vi "2DGaussianRotationModel.vi"(3 "output control":T1, 4 "data":T2, 5 "X":dbl[](array[numeric]), 6 "a":dbl[](array[numeric])) -> (0 "error out":errorcluster, 1 "f'(X,a)":dbl[][](array[numeric]), 2 "f(X,a)":dbl[](array[numeric]))   [LabVIEW 2015]
doc: "This template is the starting point for creating a model function to be passed to the Nonlinear Curve Fit.vi."
uses:
  <vilib>/gmath/NumericalOptimization/objective function data.ctl
  <vilib>/gmath/NumericalOptimization/LM_output select.ctl
  <vilib>/Analysis/baseanly.llb/A x Vector.vi
  <vilib>/Analysis/Matrix/Numeric/Conversions/Array To Matrix - RA2.vi
  <vilib>/Analysis/NI_AALBase.lvlib
  <vilib>/Analysis/Matrix/NI_Matrix.lvlib
  <vilib>/gmath/NI_Gmath.lvlib
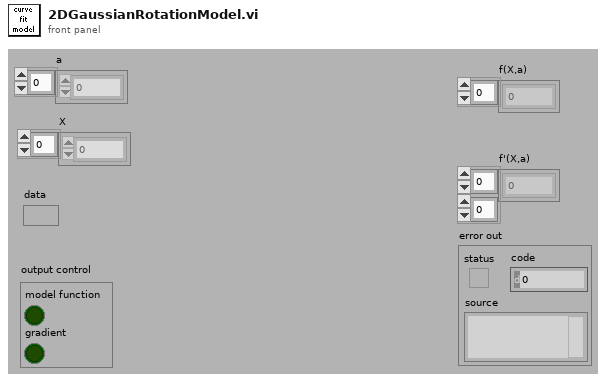
[diagram p1: front panel]
types:
  T1 = typedef "NI_Gmath.lvlib/LM_output select.ctl" = cluster{"model function":bool, "gradient":bool}
  T2 = typedef "NI_Gmath.lvlib/objective function data.ctl" = variant
  T3 = typedef "NI_Matrix.lvlib/RealMatrix.ctl" = dbl[][]
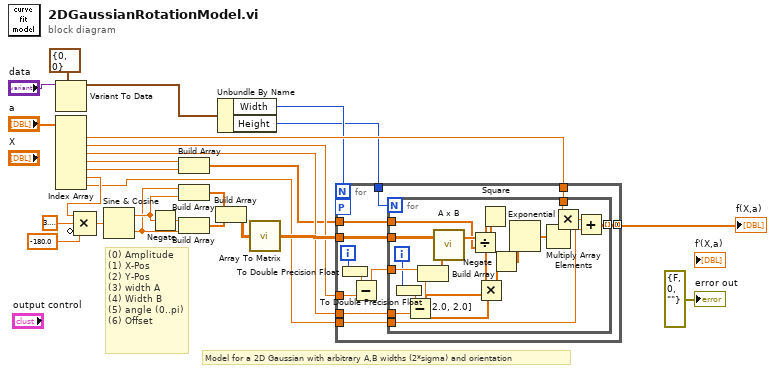
[diagram p0: block diagram]
diagram:
  # "Model for a 2D Gaussian with arbitrary A,B widths (2*sigma) and orientation"
  # "(0) Amplitude\n(1) X-Pos\n(2) Y-Pos\n(3) width A\n(4) Width B\n(5) angle (0..pi)\n(6) Offset"
  n1 = Variant To Data(type=cluster{"Width":i32, "Height":i32} {"Width"=0, "Height"=0} ("Plot Area:Size"), Variant="data") -> (data=w15:cluster{"Width":i32, "Height":i32})  [unwired: 1 in, 1 out]
  n2 = Index Array(array="a") -> (element #1=w19:dbl, element #2=w10:dbl, element #3=w9:dbl, element #4=w18:dbl, element #5=w17:dbl, element #6=w5:dbl, element #7=w4:dbl)  [unwired: 7 in]
  n3 = Compound Arithmetic op=MULTIPLY(w5, 3.141592653589793, invert -180.0 ("value")) -> (w8:dbl)
  n4 = Sine & Cosine(0:w8) -> (1:w25:dbl, 2:w24:dbl)
  n5 = Negate(x=w25) -> (-x=w26:dbl)
  n6 = Build Array(w18, w17) -> (w2:dbl[])
  n7 = Build Array(w24, w25) -> (w23:dbl[])
  n8 = Build Array(w26, w24) -> (w22:dbl[])
  n9 = Build Array(w23, w22) -> (w21:dbl[][])
  n10 = Unbundle By Name(w15) -> ("Width"=w12:i32, "Height"=w11:i32)
  n11 = call-poly <vilib>:"Array To Matrix.vi"("Real 2D Array"=w21) -> ("Real Matrix"=w20:T3)
  n12 = for {
    N: w12 -> [_]
    tunnel: w20 -> [w37]
    tunnel: w2 -> [w36]
    tunnel: [w35] -> w3 mode=concatenating
    tunnel: w19 -> [w34]
    tunnel: w11 -> [w33]
    tunnel: w10 -> [w30]
    tunnel: w9 -> [w28]
    workers-P: _ -> [_]
    tunnel: w4 -> [w27]
    i -> [w32]
    n13 = To Double Precision Float(number=w32) -> (double precision float=w31:dbl)
    n14 = Subtract(x=w31, y=w30) -> (x-y=w29:dbl)
    n15 = for {
      N: w33 -> [_]
      tunnel: w29 -> [w57]
      tunnel: w37 -> [w55]
      tunnel: w36 -> [w53]
      tunnel: [w41] -> w35 mode=indexing
      tunnel: w34 -> [w49]
      tunnel: w28 -> [w46]
      tunnel: w27 -> [w40]
      i -> [w48]
      n16 = To Double Precision Float(number=w48) -> (double precision float=w47:dbl)
      n17 = Subtract(x=w47, y=w46) -> (x-y=w45:dbl)
      n18 = Build Array(w57, w45) -> (w56:dbl[])
      n19 = call-poly <vilib>:"A x B.vi"("Vector"=w56, "A"=w55) -> ("A x Vector"=w54:dbl[])  [unwired: 1 out]
      n20 = Divide(x=w54, y=w53) -> (x/y=w44:dbl[])
      n21 = Square(x=w44) -> (x^2=w43:dbl[])
      n22 = Multiply(x=w43, y=dbl[] [2.0, 2.0]) -> (x*y=w39:dbl[])
      n23 = Negate(x=w39) -> (-x=w42:dbl[])
      n24 = Exponential(1:w42) -> (0:w52:dbl[])
      n25 = Multiply Array Elements(1:w52) -> (0:w51:dbl)
      n26 = Multiply(x=w49, y=w51) -> (x*y=w50:dbl)
      n27 = Add(x=w50, y=w40) -> (x+y=w41:dbl)
    }
  }
  "f(X,a)" <- w3
  "error out" <- errorcluster {"status"=FALSE, "code"=0, "source"=""} ("error out")
